vi "Simulated VeriStand Engine.Create.vi"(8 "error in (no error)":errorcluster, 10 "Simulated Custom Devices":refnum<class "Simulated VeriStand Custom Device.lvclass">[](array[class]), 11 "Simulated VeriStand Engine in":refnum<class "Simulated VeriStand Engine.lvclass">) -> (0 "error out":errorcluster, 3 "Simulated VeriStand Engine out":refnum<class "Simulated VeriStand Engine.lvclass">)   [LabVIEW 2016, in "Simulated VeriStand Engine.lvclass"]
uses:
  Simulated VeriStand Engine.lvclass
  Simulated VeriStand Custom Device/Simulated VeriStand Custom Device.lvclass
  Simulated VeriStand Engine Interface/Simulated VeriStand Engine.Interface.lvclass/Simulated VeriStand Engine.Interface.ctl
  Simulated VeriStand Engine.lvclass/Simulated VeriStand Engine.ctl
  Simulated VeriStand Engine Interface/Methods/Simulated VeriStand Engine.Interface.Allocate.Status Pointers.vi
  Simulated VeriStand Engine Interface/Methods/Simulated VeriStand Engine.Interface.Allocate.Control Pointers.vi
  Source/Submodules/Memory/Source/Classes/Internal/Memory.Pointer.Internal.New.vi
  Simulated VeriStand Engine Interface/Accessors/Simulated VeriStand Engine.Interface.Set Status Pointers.vi
  Simulated VeriStand Engine Interface/Accessors/Simulated VeriStand Engine.Interface.Set Control Pointers.vi
  Source/Submodules/Memory/Source/Classes/Internal/Memory.Pointer.Internal.Allocate.vi
  Source/Submodules/Memory/Source/Classes/Internal/Memory.Pointer.Internal.lvclass
  Simulated VeriStand Engine Interface/Simulated VeriStand Engine.Interface.lvclass
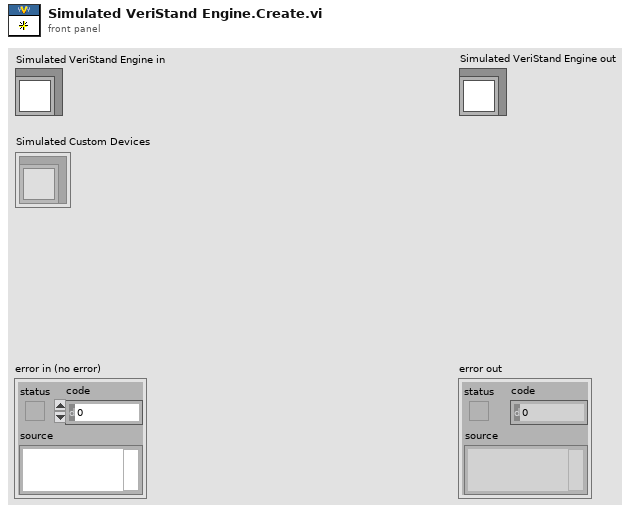
[diagram p1: front panel]
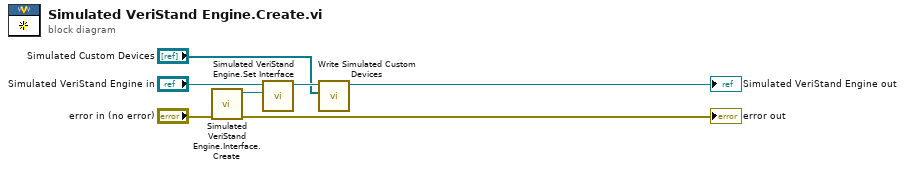
[diagram p0: block diagram]
diagram:
  n1 = call "Simulated VeriStand Engine.Interface.Create.vi"("error in (no error)"="error in (no error)") -> ("error out"=→"error out":errorcluster, "Simulated VeriStand Engine Interface out"=w6:refnum<class "Simulated VeriStand Engine.Interface.lvclass">)  [unwired: 9 in]
  n2 = call "Simulated VeriStand Engine.Set Interface.vi"("Interface"=w6, "Simulated VeriStand Engine in"="Simulated VeriStand Engine in") -> ("Simulated VeriStand Engine out"=w4:refnum<class "Simulated VeriStand Engine.lvclass">)  [unwired: 8 in, 1 out]
  n3 = call "Write Simulated Custom Devices.vi"("Simulated Custom Devices"="Simulated Custom Devices", "Simulated VeriStand Engine in"=w4) -> ("Simulated VeriStand Engine out"=→"Simulated VeriStand Engine out":refnum<class "Simulated VeriStand Engine.lvclass">)  [unwired: 8 in, 1 out]
